vi "Fast Get Multiple Dependent Node Refs FuncGlobal.vi"(5 "Action":T1(ring), 8 "error in (no error)":errorcluster, 10 "Base Property Name":string, 11 "Item Ref in":T2 format="%.0x") -> (0 "error out":errorcluster, 1 "Dependent Node Refs":T2[](array[typedef]) format="%.0x", 3 "Item Ref out":T2=18446744073709551615 format="%.0x")   [LabVIEW 2011]
uses:
  <vilib>/NI Veristand/Custom Device API/Custom Device Item Ref.ctl
  <vilib>/NI Veristand/Custom Device API/Get Item Property (Variant).vi
  <vilib>/NI Veristand/Custom Device API/Set Item Property (Variant).vi
  <vilib>/NI Veristand/Custom Device API/Custom Device API.lvlib
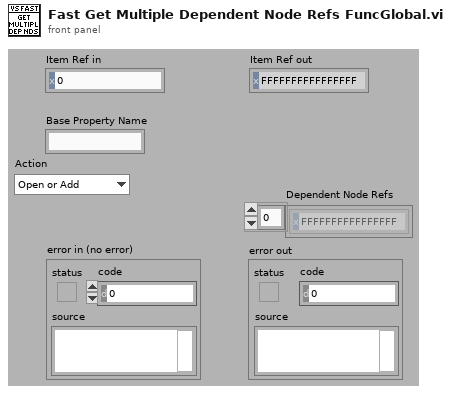
[diagram p1: front panel]
types:
  T1 = enum16{"Open or Add", "Close Ref", "Reset Local Store"}
  T2 = typedef "Custom Device API.lvlib/Custom Device Item Ref.ctl" = u64
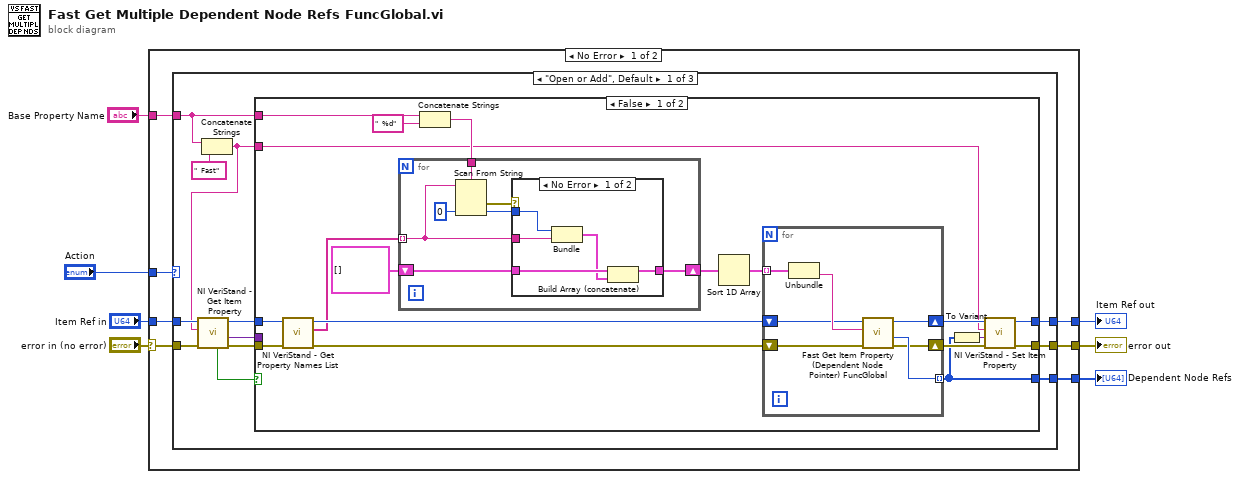
[diagram p0: block diagram]
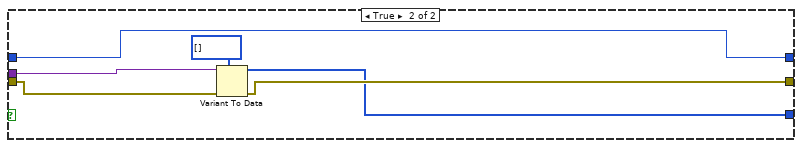
[diagram p3: hidden frame]
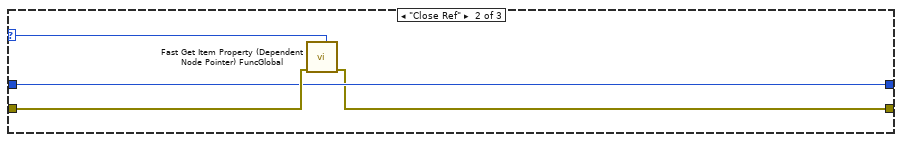
[diagram p4: hidden frame]
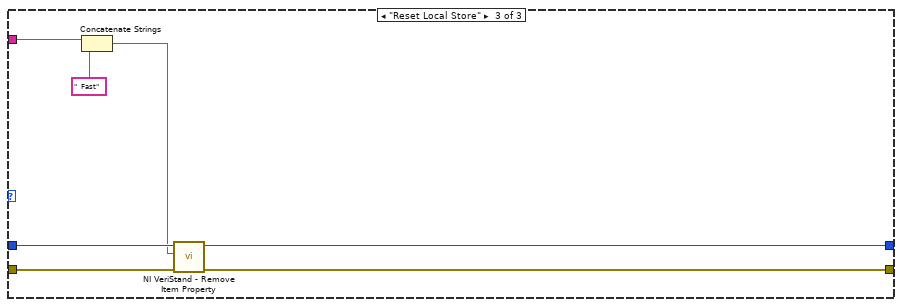
[diagram p5: hidden frame]
diagram:
  n1 = case shown="No Error" "error in (no error)" {
    selector: "error in (no error)" -> [w12 w82]
    tunnel: "Item Ref in" -> [w14 w83]
    tunnel: [w11 w83] -> w6
    tunnel: [w10 w82] -> w5
    tunnel: "Base Property Name" -> [w13 _]
    tunnel: [w9 _] -> w2
    tunnel: "Action" -> [w8 _]
    frame No Error {
      n2 = case shown="\"Open or Add\", Default" w8 {
        selector: w8 -> [_ w74 _]
        tunnel: w14 -> [w20 w72 w79]
        tunnel: w13 -> [w17 _ w80]
        tunnel: w12 -> [w23 w73 w78]
        tunnel: [w26 w72 w75] -> w11
        tunnel: [w25 w71 w76] -> w10
        tunnel: [w24 _ _] -> w9
        frame "Open or Add", Default {
          n3 = Concatenate Strings(w17, "  Fast" ("string")) -> (w15:string)
          n4 = call-poly <vilib>:"NI VeriStand - Get Item Property.vi"("error in (no error)"=w23, "Property Name"=w15, "Item Ref in"=w20) -> ("error out"=w22:errorcluster, "Value"=w18:variant, "Item Ref out"=w21:T2, "Found?"=w19:bool)  [unwired: 5 in]
          n5 = case shown="False" w19 {
            tunnel: w17 -> [w44 _]
            tunnel: [w32 w65] -> w26
            tunnel: [w30 w67] -> w25
            tunnel: [w27 w66] -> w24
            tunnel: w22 -> [w35 w68]
            tunnel: w21 -> [w34 w65]
            tunnel: w18 -> [_ w69]
            tunnel: w15 -> [w29 _]
            frame False {
              n6 = call <vilib>:"NI VeriStand - Get Property Names List.vi"("error in (no error)"=w35, "Item Ref in"=w34) -> ("error out"=w38:errorcluster, "Property Names"=w36:string[], "Item Ref out"=w39:T2)  [unwired: 7 in]
              n7 = Concatenate Strings(w44, "  %d" ("string")) -> (w42:string)
              n8 = for {
                tunnel: w36 -> [w57] mode=indexing
                tunnel: w42 -> [w56]
                shift-right: [w53] -> w40
                shift-left: cluster{"default value 1":i32, string}[] [] -> [w52]
                n9 = Scan From String(format string=w56, input string=w57, default 1=0 ("default value 1")) -> (error out=w58:errorcluster, output 1=w54:i32)  [unwired: 2 in, 2 out]
                n10 = case shown="No Error" w58 {
                  tunnel: w57 -> [w62 _]
                  tunnel: w54 -> [w63 _]
                  tunnel: [w61 w64] -> w53
                  tunnel: w52 -> [w60 w64]
                  frame No Error {
                    n11 = Bundle("default value 1"=w63, w62) -> (w59:cluster{"default value 1":i32, string})  [unwired: 1 in]
                    n12 = Build Array (concatenate)(w60, w59) -> (w61:cluster{"default value 1":i32, string}[])
                  }
                  frame Error {
                  }
                }
              }
              n13 = Sort 1D Array(array=w40) -> (sorted array=w37:cluster{"default value 1":i32, string}[])
              n14 = for {
                shift-right: [w47] -> w33
                shift-left: w39 -> [w48]
                shift-right: [w45] -> w31
                shift-left: w38 -> [w50]
                tunnel: w37 -> [w51] mode=indexing
                tunnel: [w46] -> w27 mode=indexing
                n15 = Unbundle(w51) -> (w49:string)  [unwired: 1 out]
                n16 = call "Fast Get Item Property (Dependent Node Pointer) FuncGlobal.vi"("error in (no error)"=w50, "Property Name"=w49, "Item Ref in"=w48) -> ("error out"=w45:errorcluster, "Dependent Node Ref"=w46:T2, "Item Ref out"=w47:T2)  [unwired: 5 in, 1 out]
              }
              n17 = To Variant(anything=w27) -> (Variant=w28:variant)
              n18 = call-poly <vilib>:"NI VeriStand - Set Item Property.vi"("error in (no error)"=w31, "Value"=w28, "Property Name"=w29, "Item Ref in"=w33) -> ("error out"=w30:errorcluster, "Item Ref out"=w32:T2)  [unwired: 5 in, 1 out]
            }
            frame True {
              n19 = Variant To Data(error in=w68, type=T2[] [], Variant=w69) -> (data=w66:T2[], error out=w67:errorcluster)
            }
          }
        }
        frame "Close Ref" {
          n20 = call "Fast Get Item Property (Dependent Node Pointer) FuncGlobal.vi"("Action"=w74, "error in (no error)"=w73) -> ("error out"=w71:errorcluster)  [unwired: 6 in, 3 out]
        }
        frame "Reset Local Store" {
          n21 = Concatenate Strings(w80, "  Fast" ("string")) -> (w77:string)
          n22 = call <vilib>:"NI VeriStand - Remove Item Property.vi"("error in (no error)"=w78, "Property Name"=w77, "Item Ref in"=w79) -> ("error out"=w76:errorcluster, "Item Ref out"=w75:T2)  [unwired: 6 in, 1 out]
        }
      }
    }
    frame Error {
    }
  }
  "Dependent Node Refs" <- w2
  "Item Ref out" <- w6
  "error out" <- w5
